vi "convert_string_to_int64.vi"(3 "default (0)":i64, 4 "String in":string) -> (1 "int64 value out":i64)   [LabVIEW 2020, in "Rohde&Schwarz RTx Oscilloscopes.lvlib" / "rsidr_core.lvlib"]
uses:
  rsidr_core.lvlib
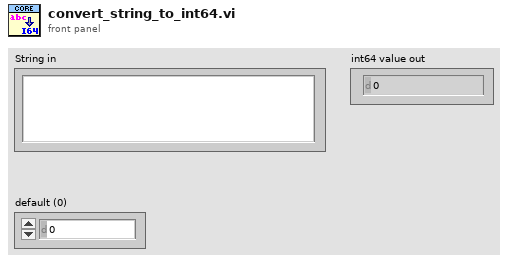
[diagram p1: front panel]
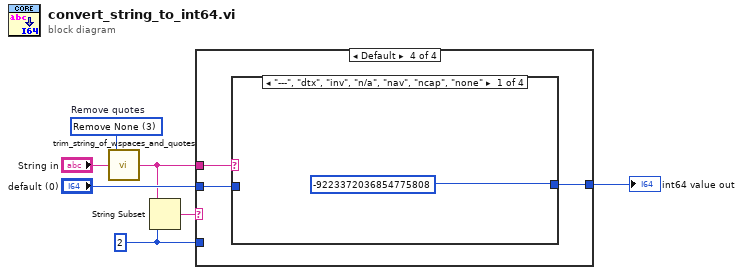
[diagram p0: block diagram]
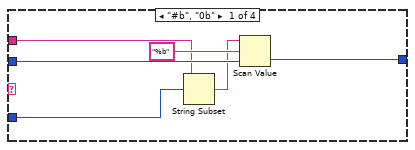
[diagram p2: hidden frame]
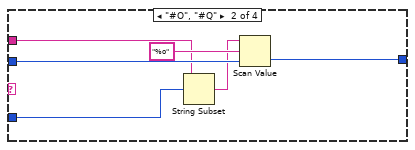
[diagram p3: hidden frame]
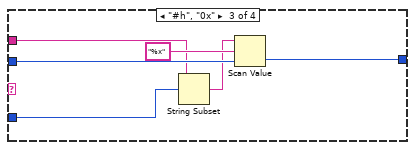
[diagram p4: hidden frame]
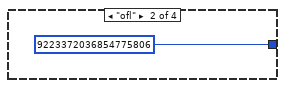
[diagram p5: hidden frame]
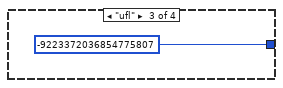
[diagram p6: hidden frame]
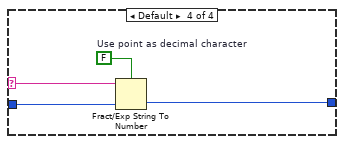
[diagram p7: hidden frame]
diagram:
  w3 = u16 3 items=["Remove All Quotes", "Remove Single Quotes", "Remove Double Quotes", "Remove None"]  # Remove quotes
  w6 = 2 ("length (rest)")
  n1 = call "trim_string_of_wspaces_and_quotes.vi"("String in"="String in", "Remove quotes (Remove All)"=w3) -> ("String out"=w1:string)  [unwired: 3 in]
  n2 = String Subset(string=w1, length (rest)=w6) -> (substring=w7:string)  [unwired: 1 in]
  n3 = case shown="Default" w7 {
    tunnel: [w13 w19 w25 w26] -> w4
    tunnel: w1 -> [w9 w15 w21 w28]
    tunnel: "default (0)" -> [w12 w18 w24 w27]
    tunnel: w6 -> [w10 w16 w22 _]
    frame "#b", "0b" {
      n4 = String Subset(string=w9, offset (0)=w10) -> (substring=w8:string)  [unwired: 1 in]
      n5 = Scan Value(string=w8, format string="%b", default (0 dbl)=w12) -> (value=w13:i64)  [unwired: 1 out]
    }
    frame "#O", "#Q" {
      n6 = String Subset(string=w15, offset (0)=w16) -> (substring=w14:string)  [unwired: 1 in]
      n7 = Scan Value(string=w14, format string="%o", default (0 dbl)=w18) -> (value=w19:i64)  [unwired: 1 out]
    }
    frame "#h", "0x" {
      n8 = String Subset(string=w21, offset (0)=w22) -> (substring=w20:string)  [unwired: 1 in]
      n9 = Scan Value(string=w20, format string="%x", default (0 dbl)=w24) -> (value=w25:i64)  [unwired: 1 out]
    }
    frame Default {
      n10 = case shown="\"---\", \"dtx\", \"inv\", \"n/a\", \"nav\", \"ncap\", \"none\"" w28 {
        selector: w28 -> [_ _ _ w32]
        tunnel: w27 -> [_ _ _ w35]
        tunnel: [i64 -9223372036854775808 i64 9223372036854775806 i64 -9223372036854775807 w34] -> w26
        frame "---", "dtx", "inv", "n/a", "nav", "ncap", "none" {
        }
        frame "ofl" {
        }
        frame "ufl" {
        }
        frame Default {
          w33 = FALSE  # Use point as decimal character
          n11 = Fract/Exp String To Number(use system decimal point (T)=w33, string=w32, default (0 dbl)=w35) -> (number=w34:i64)  [unwired: 1 in, 1 out]
        }
      }
    }
  }
  "int64 value out" <- w4
